vi "Bounding Box to Rectangle.vi"(8 "Error In":errorcluster, 11 "Bounding Box":T1) -> (0 "Error Out":errorcluster, 3 "Rectangle":i32[](array[numeric]))   [LabVIEW 2018]
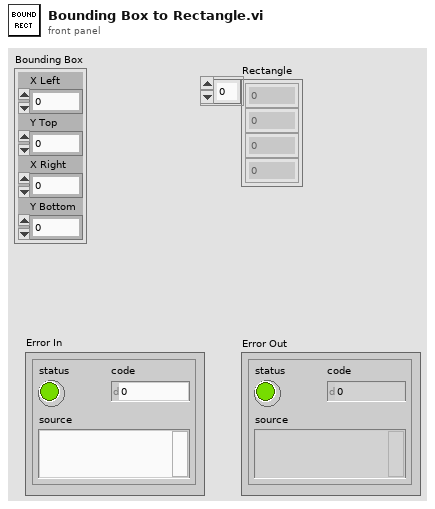
[diagram p1: front panel]
types:
  T1 = cluster{"X Left":i32, "Y Top":i32, "X Right":i32, "Y Bottom":i32}
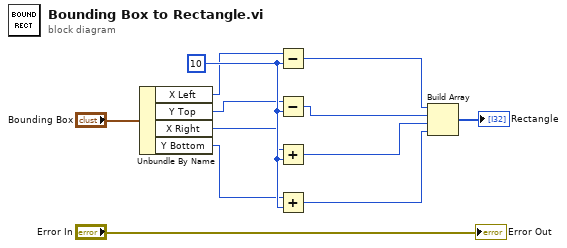
[diagram p0: block diagram]
diagram:
  w11 = 10
  n1 = Unbundle By Name("Bounding Box") -> ("X Left"=w10:i32, "Y Top"=w9:i32, "X Right"=w8:i32, "Y Bottom"=w7:i32)
  n2 = Subtract(x=w10, y=w11) -> (x-y=w6:i32)
  n3 = Subtract(x=w9, y=w11) -> (x-y=w5:i32)
  n4 = Add(x=w8, y=w11) -> (x+y=w4:i32)
  n5 = Add(x=w7, y=w11) -> (x+y=w3:i32)
  n6 = Build Array(w6, w5, w4, w3) -> (→"Rectangle":i32[])
  "Error Out" <- "Error In"
